vi "putForceActuatorStatus.vi"(8 "error in (no error)":errorcluster, 10 "TelemetryForceActuatorStatus":T1, 11 "M1M3SAL in":refnum<class "M1M3SAL.lvclass">) -> (0 "error out":errorcluster, 3 "M1M3SAL out":refnum<class "M1M3SAL.lvclass">)   [LabVIEW 2016, in "M1M3SupportCommunicator.lvlib" / "M1M3SAL.lvclass"]
uses:
  M1M3SAL.lvclass
  DataTypes/Topics/TelemetryForceActuatorStatus.ctl
  DataTypes/Topics/Parts/Timestamp.ctl
  DataTypes/MessageHeader.ctl
  DataTypes/MessageTypes.ctl
  DataTypes/MessageTopics.ctl
  M1M3SAL.lvclass/M1M3SAL.ctl
  writeU8.vi
  writeI32.vi
  writeBoolean.vi
  M1M3SupportCommunicator.lvlib
  DataTypes/Topics/M1M3SupportTopics.lvlib
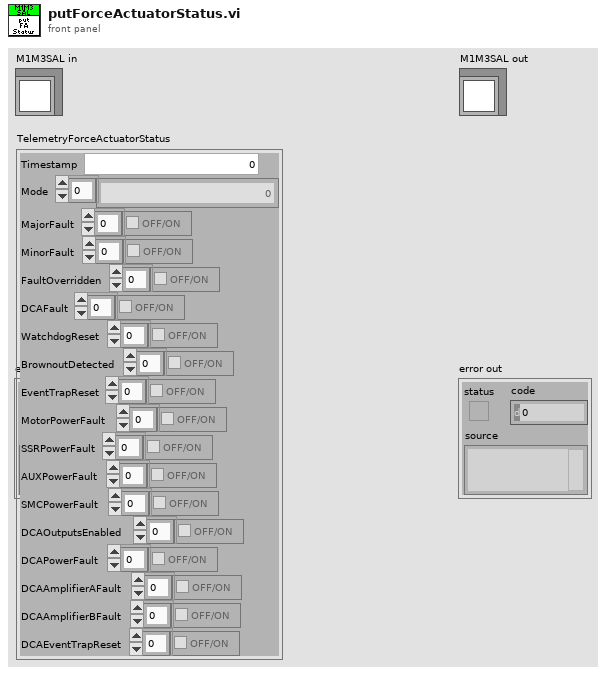
[diagram p1: front panel]
types:
  T1 = typedef "M1M3SupportTopics.lvlib/TelemetryForceActuatorStatus.ctl" = cluster{"Timestamp":T2, "Mode":u8[], "MajorFault":bool[], "MinorFault":bool[], "FaultOverridden":bool[], "DCAFault":bool[], "WatchdogReset":bool[], "BrownoutDetected":bool[], "EventTrapReset":bool[], "MotorPowerFault":bool[], "SSRPowerFault":bool[], "AUXPowerFault":bool[], "SMCPowerFault":bool[], "DCAOutputsEnabled":bool[], "DCAPowerFault":bool[], "DCAAmplifierAFault":bool[], "DCAAmplifierBFault":bool[], "DCAEventTrapReset":bool[]}
  T2 = typedef "M1M3SupportTopics.lvlib/Timestamp.ctl" = dbl
  T3 = typedef "M1M3SupportCommunicator.lvlib/MessageHeader.ctl" = cluster{"Type":T4, "Topic":T5, "Size":i32}
  T4 = typedef "M1M3SupportCommunicator.lvlib/MessageTypes.ctl" = enum8{"None", "PutSample", "GetNextSample", "LogEvent", "GetEvent", "IssueCommand", "CommandId", "WaitForCompletion", "AcceptCommand", "AckCommand"}
  T5 = typedef "M1M3SupportCommunicator.lvlib/MessageTopics.ctl" = enum8{"None", "ForceActuatorData", "MirrorForceData", "HardpointData", "AirData", "DynamicData", "FPGAData", "IMSData", "ForceActuatorStatus", "ElevationData", "HardpointStatus", "HardpointActuatorChase", "AirStatus", "ForceActuatorSafetyChecks", "ForceActuatorTest", "ActuatorBroadcastCounter", "StatusChecks", "CellChecks", "HardpointActuatorBreakaway", "RaiseMirrorComplete", "ILCCommunication", "ElevationAngleChecks", "DetailedState", "ServoLoops", "ForceActuatorInfo", "LowerMirrorComplete", "HardpointActuatorInfo", "SettingsApplied", "ErrorCode", "StartupChecks", "SummaryState", "SettingVersions", "ActuatorTestStatus", "AppliedSettingsMatchStart", "Enable", "EnterMaintenance", "Standby", "AbortLowerM1M3", "ApplyAberrationByForces", "ApplyAOSCorrectionByBendingModes", "ClearAOSCorrection", "Start", "RaiseM1M3", "TestForceActuator", "LowerM1M3", "ApplyAOSCorrectionByForces", "Disable", "ApplyAberationByBendingMode", "TestHardpoint", "ManipulateM1M3", "ClearAberration", "Exit", "TestAir", "AbortRaiseM1M3", "MoveHardpointActuators", "ExitMaintenance", "Shutdown"}
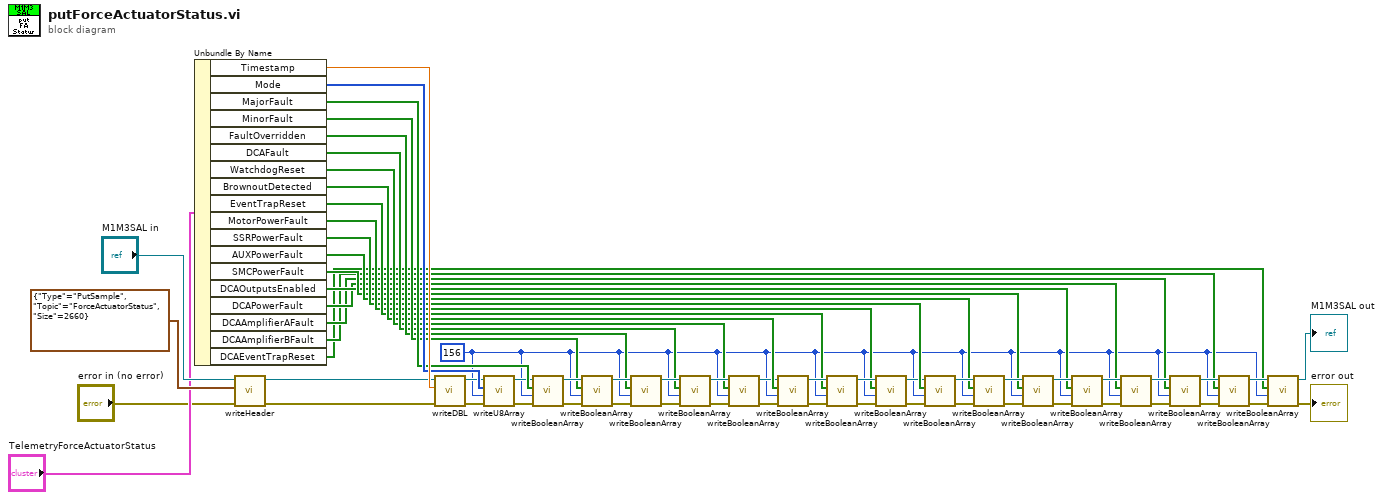
[diagram p0: block diagram]
diagram:
  w1 = 156 ("Length")
  n1 = Unbundle By Name("TelemetryForceActuatorStatus") -> ("Timestamp"=w46:T2, "Mode"=w45:u8[], "MajorFault"=w44:bool[], "MinorFault"=w43:bool[], "FaultOverridden"=w42:bool[], "DCAFault"=w41:bool[], "WatchdogReset"=w40:bool[], "BrownoutDetected"=w39:bool[], "EventTrapReset"=w38:bool[], "MotorPowerFault"=w37:bool[], "SSRPowerFault"=w36:bool[], "AUXPowerFault"=w25:bool[], "SMCPowerFault"=w24:bool[], "DCAOutputsEnabled"=w23:bool[], "DCAPowerFault"=w22:bool[], "DCAAmplifierAFault"=w21:bool[], "DCAAmplifierBFault"=w16:bool[], "DCAEventTrapReset"=w15:bool[])
  n2 = call "writeHeader.vi"("error in (no error)"="error in (no error)", "MessageHeader"=T3 {"Type"=enum."PutSample", "Topic"=enum."ForceActuatorStatus", "Size"=2660}, "M1M3SAL in"="M1M3SAL in") -> ("error out"=w10:errorcluster, "M1M3SAL out"=w14:refnum<class "M1M3SAL.lvclass">)  [unwired: 7 in]
  n3 = call "writeDBL.vi"("error in (no error)"=w10, "Input"=w46, "M1M3SAL in"=w14) -> ("error out"=w9:errorcluster, "M1M3SAL out"=w13:refnum<class "M1M3SAL.lvclass">)  [unwired: 7 in]
  n4 = call "writeU8Array.vi"("error in (no error)"=w9, "Length"=w1, "Input"=w45, "M1M3SAL in"=w13) -> ("error out"=w8:errorcluster, "M1M3SAL out"=w12:refnum<class "M1M3SAL.lvclass">)  [unwired: 6 in]
  n5 = call "writeBooleanArray.vi"("error in (no error)"=w8, "Length"=w1, "Input"=w44, "M1M3SAL in"=w12) -> ("error out"=w58:errorcluster, "M1M3SAL out"=w57:refnum<class "M1M3SAL.lvclass">)  [unwired: 6 in]
  n6 = call "writeBooleanArray.vi"("error in (no error)"=w58, "Length"=w1, "Input"=w43, "M1M3SAL in"=w57) -> ("error out"=w56:errorcluster, "M1M3SAL out"=w55:refnum<class "M1M3SAL.lvclass">)  [unwired: 6 in]
  n7 = call "writeBooleanArray.vi"("error in (no error)"=w56, "Length"=w1, "Input"=w42, "M1M3SAL in"=w55) -> ("error out"=w54:errorcluster, "M1M3SAL out"=w53:refnum<class "M1M3SAL.lvclass">)  [unwired: 6 in]
  n8 = call "writeBooleanArray.vi"("error in (no error)"=w54, "Length"=w1, "Input"=w41, "M1M3SAL in"=w53) -> ("error out"=w52:errorcluster, "M1M3SAL out"=w51:refnum<class "M1M3SAL.lvclass">)  [unwired: 6 in]
  n9 = call "writeBooleanArray.vi"("error in (no error)"=w52, "Length"=w1, "Input"=w40, "M1M3SAL in"=w51) -> ("error out"=w3:errorcluster, "M1M3SAL out"=w4:refnum<class "M1M3SAL.lvclass">)  [unwired: 6 in]
  n10 = call "writeBooleanArray.vi"("error in (no error)"=w3, "Length"=w1, "Input"=w39, "M1M3SAL in"=w4) -> ("error out"=w50:errorcluster, "M1M3SAL out"=w49:refnum<class "M1M3SAL.lvclass">)  [unwired: 6 in]
  n11 = call "writeBooleanArray.vi"("error in (no error)"=w50, "Length"=w1, "Input"=w38, "M1M3SAL in"=w49) -> ("error out"=w48:errorcluster, "M1M3SAL out"=w47:refnum<class "M1M3SAL.lvclass">)  [unwired: 6 in]
  n12 = call "writeBooleanArray.vi"("error in (no error)"=w48, "Length"=w1, "Input"=w37, "M1M3SAL in"=w47) -> ("error out"=w7:errorcluster, "M1M3SAL out"=w11:refnum<class "M1M3SAL.lvclass">)  [unwired: 6 in]
  n13 = call "writeBooleanArray.vi"("error in (no error)"=w7, "Length"=w1, "Input"=w36, "M1M3SAL in"=w11) -> ("error out"=w35:errorcluster, "M1M3SAL out"=w34:refnum<class "M1M3SAL.lvclass">)  [unwired: 6 in]
  n14 = call "writeBooleanArray.vi"("error in (no error)"=w35, "Length"=w1, "Input"=w25, "M1M3SAL in"=w34) -> ("error out"=w33:errorcluster, "M1M3SAL out"=w32:refnum<class "M1M3SAL.lvclass">)  [unwired: 6 in]
  n15 = call "writeBooleanArray.vi"("error in (no error)"=w33, "Length"=w1, "Input"=w24, "M1M3SAL in"=w32) -> ("error out"=w31:errorcluster, "M1M3SAL out"=w30:refnum<class "M1M3SAL.lvclass">)  [unwired: 6 in]
  n16 = call "writeBooleanArray.vi"("error in (no error)"=w31, "Length"=w1, "Input"=w23, "M1M3SAL in"=w30) -> ("error out"=w26:errorcluster, "M1M3SAL out"=w27:refnum<class "M1M3SAL.lvclass">)  [unwired: 6 in]
  n17 = call "writeBooleanArray.vi"("error in (no error)"=w26, "Length"=w1, "Input"=w22, "M1M3SAL in"=w27) -> ("error out"=w29:errorcluster, "M1M3SAL out"=w28:refnum<class "M1M3SAL.lvclass">)  [unwired: 6 in]
  n18 = call "writeBooleanArray.vi"("error in (no error)"=w29, "Length"=w1, "Input"=w21, "M1M3SAL in"=w28) -> ("error out"=w20:errorcluster, "M1M3SAL out"=w19:refnum<class "M1M3SAL.lvclass">)  [unwired: 6 in]
  n19 = call "writeBooleanArray.vi"("error in (no error)"=w20, "Length"=w1, "Input"=w16, "M1M3SAL in"=w19) -> ("error out"=w18:errorcluster, "M1M3SAL out"=w17:refnum<class "M1M3SAL.lvclass">)  [unwired: 6 in]
  n20 = call "writeBooleanArray.vi"("error in (no error)"=w18, "Length"=w1, "Input"=w15, "M1M3SAL in"=w17) -> ("error out"=→"error out":errorcluster, "M1M3SAL out"=→"M1M3SAL out":refnum<class "M1M3SAL.lvclass">)  [unwired: 6 in]
